vi "AMB_CAN_Find_Slaves.vi"(0 "ObjHandle in":u32, 1 "error in":errorcluster {"code" format="%.0x"}) -> (2 "ObjHandle out":u32, 3 "NumSlaves out":u8, 4 "Node Array out":cluster{"Address":u32, "Serial Number":i8[]}[](array[cluster]) {"Serial Number" format="%.0x"}, 5 "error out":errorcluster {"code" format="%.0x"})   [LabVIEW 2017]
doc: "This VI finds all of the AMB slaves currently active on the CAN network.\nYou should have already setup the AMB with the AMB Setup VI."
panel:
  out "Temp Node":cluster{"Address":u32, "Serial Number":i8[]} {"Serial Number" format="%.0x"}
  # "ALMA Monitor and Control Bus\nFind Slave Nodes"
  # "Node Address"
  # "Serial Number"
  # "Node Address"
  # "Serial Number"
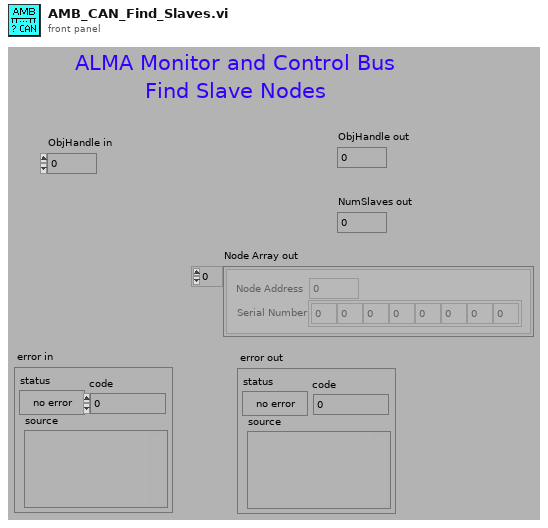
[diagram p1: front panel]
types:
  T1 = typedef "xobjhandle.ctl" = u32
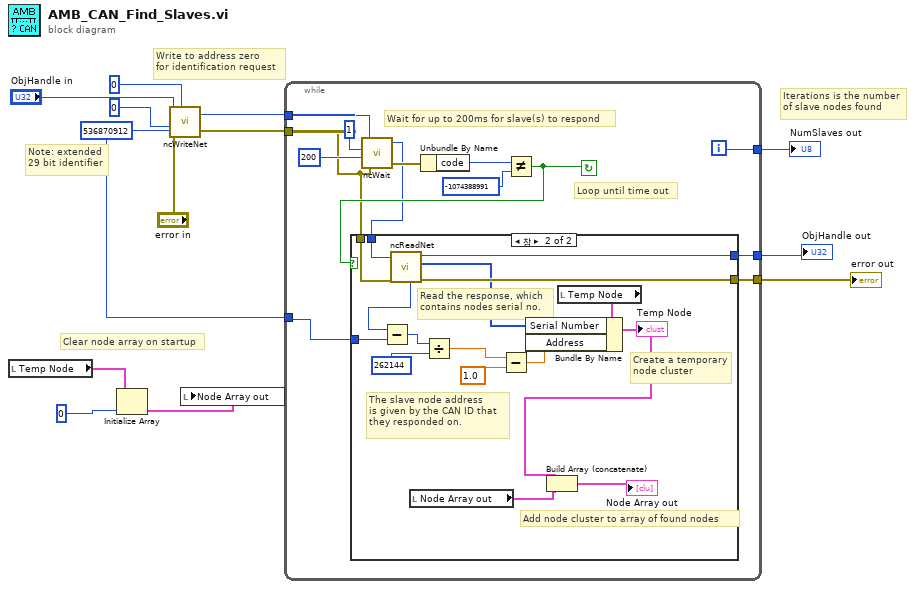
[diagram p0: block diagram]
diagram:
  w11 = u32 536870912 ("ArbitrationId")
  # "Iterations is the number\nof slave nodes found"
  # "Note: extended\n29 bit identifier"
  # "Write to address zero\nfor identification request"
  # "Clear node array on startup"
  n1 = local read "Temp Node"() -> (w7:cluster{"Address":u32, "Serial Number":i8[]})
  n2 = Initialize Array(w7, 0 ("Dimension Size")) -> (w1:cluster{"Address":u32, "Serial Number":i8[]}[])
  n3 = call <vilib>:"ncWriteNet.vi"("ArbitrationId"=w11, "DataLength"=u32 0, "Error in"="error in", "IsRemote"=u8 0, "ObjHandle in"="ObjHandle in") -> ("Error out"=w9:errorcluster, "ObjHandle out"=w10:T1)  [unwired: 1 in]
  n4 = local write "Node Array out"(w1) -> ()
  n5 = while {
    tunnel: [w15] -> w3
    tunnel: [w16] -> w2
    tunnel: w11 -> [w14]
    tunnel: [w23] -> w4
    tunnel: w9 -> [w17]
    tunnel: w10 -> [w26]
    i -> [w23]
    stop <- w19 continue-if-true
    # "Loop until time out"
    # "Wait for up to 200ms for slave(s) to respond"
    n6 = call <vilib>:"ncWait.vi"("Error in"=w17, "Timeout"=200, "DesiredState"=u32 1, "ObjHandle in"=w26) -> ("Error out"=w22:errorcluster, "ObjHandle out"=w18:T1)  [unwired: 1 out]
    n7 = Unbundle By Name(w22) -> ("code"=w21:i32)
    n8 = Not Equal?(x=w21, y=-1074388991) -> (x != y?=w19:bool)
    n9 = case shown="참" w19 {
      tunnel: w18 -> [w28 w44]
      tunnel: w17 -> [w27 w43]
      tunnel: [w28 w42] -> w16
      tunnel: [w27 w41] -> w15
      tunnel: w14 -> [_ w39]
      frame False {
        # "Timed out, we are going to exit the while loop."
      }
      frame True {
        # "Add node cluster to array of found nodes"
        # "Create a temporary\nnode cluster"
        # "The slave node address\nis given by the CAN ID that\nthey responded on."
        # "Read the response, which\ncontains nodes serial no."
        n10 = call <vilib>:"ncReadNet.vi"("ObjHandle in"=w44, "Error in"=w43) -> ("ArbitrationId"=w40:u32, "ObjHandle out"=w42:T1, "Data"=w34:u8[], "Error out"=w41:errorcluster)  [unwired: 2 in, 3 out]
        n11 = Subtract(x=w40, y=w39) -> (x-y=w38:u32)
        n12 = local read "Node Array out"() -> (w29:cluster{"Address":u32, "Serial Number":i8[]}[])
        n13 = Divide(x=w38, y=u32 262144) -> (x/y=w36:dbl)
        n14 = Subtract(x=w36, y=1.0) -> (x-y=w33:dbl)
        n15 = local read "Temp Node"() -> (w32:cluster{"Address":u32, "Serial Number":i8[]})
        n16 = Bundle By Name(cluster=w32, "Serial Number"=w34, "Address"=w33) -> (w30:cluster{"Address":u32, "Serial Number":i8[]})
        "Temp Node" <- w30
        n17 = Build Array (concatenate)(w30, w29) -> (→"Node Array out":cluster{"Address":u32, "Serial Number":i8[]}[])
      }
    }
  }
  "error out" <- w3
  "ObjHandle out" <- w2
  "NumSlaves out" <- w4
